vi "Cold_Flow_Test.vi"() -> ()   [LabVIEW 2024]
panel:
  in  "Stop":bool
  in  "Flow Time, ms":u32=1000
  out "Kerosene Valve":bool
  out "GOX Valve":bool
  in  "GOX Channel":tag="Dev1/port0/line1"
  in  "Kerosene Channel":tag="Dev1/port0/line3"
  # "Cold Flow Torch Igniter Test"
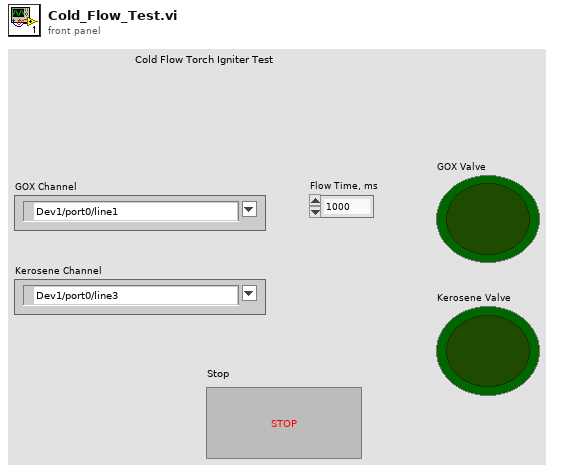
[diagram p1: front panel]
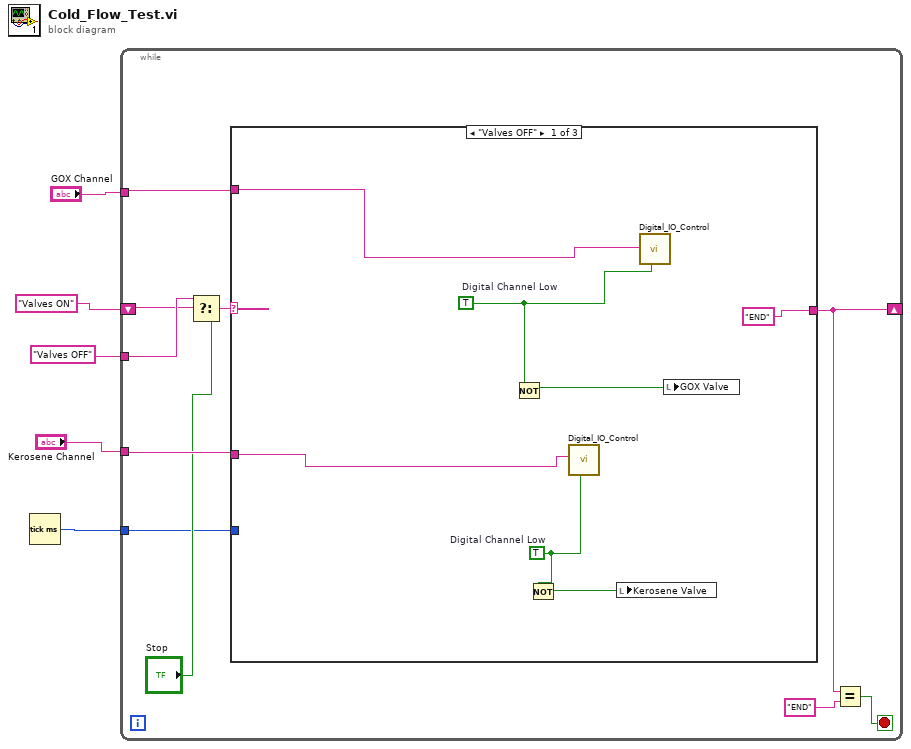
[diagram p0: block diagram]
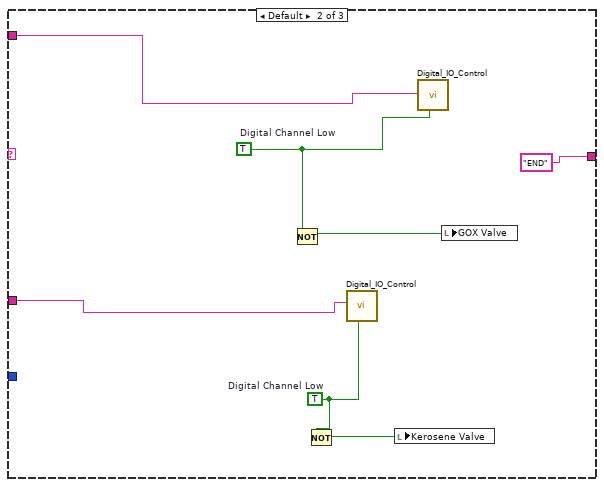
[diagram p2: hidden frame]
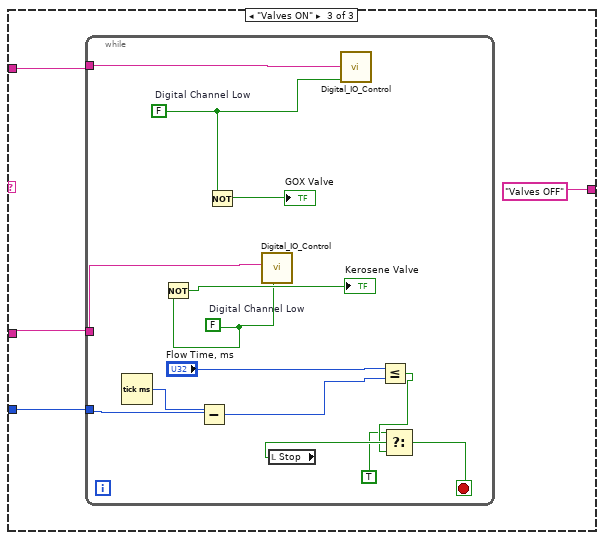
[diagram p3: hidden frame]
diagram:
  n1 = Tick Count (ms)() -> (millisecond timer value=w1:u32)
  n2 = while {
    tunnel: "Valves OFF" -> [w12]
    shift-right: [w8] -> _
    shift-left: "Valves ON" -> [w11]
    tunnel: "GOX Channel" -> [w15]
    tunnel: "Kerosene Channel" -> [w14]
    tunnel: w1 -> [w6]
    stop <- w9 stop-if-true
    n3 = Select(t=w12, s="Stop", f=w11) -> (s? t:f=w13:string)
    n4 = case shown="\"Valves OFF\"" w13 {
      tunnel: w15 -> [w20 w27 w33]
      tunnel: w14 -> [w19 w26 w32]
      tunnel: ["END" "END" "Valves OFF"] -> w8
      tunnel: w6 -> [_ _ w30]
      frame "Valves OFF" {
        w21 = TRUE  # Digital Channel Low
        w22 = TRUE  # Digital Channel Low
        n5 = Not(x=w22) -> (.not. x?=w18:bool)
        n6 = Not(x=w21) -> (.not. x?=w17:bool)
        n7 = call "Digital_IO_Control.vi"("Digital Channel High/Low (false : low)"=w21, "Digital Port Seclection"=w19) -> ()  [unwired: 6 in, 1 out]
        n8 = local write "Kerosene Valve"(w17) -> ()
        n9 = call "Digital_IO_Control.vi"("Digital Channel High/Low (false : low)"=w22, "Digital Port Seclection"=w20) -> ()  [unwired: 6 in, 1 out]
        n10 = local write "GOX Valve"(w18) -> ()
      }
      frame Default {
        w28 = TRUE  # Digital Channel Low
        w29 = TRUE  # Digital Channel Low
        n11 = Not(x=w29) -> (.not. x?=w25:bool)
        n12 = Not(x=w28) -> (.not. x?=w24:bool)
        n13 = call "Digital_IO_Control.vi"("Digital Channel High/Low (false : low)"=w28, "Digital Port Seclection"=w26) -> ()  [unwired: 6 in, 1 out]
        n14 = local write "Kerosene Valve"(w24) -> ()
        n15 = call "Digital_IO_Control.vi"("Digital Channel High/Low (false : low)"=w29, "Digital Port Seclection"=w27) -> ()  [unwired: 6 in, 1 out]
        n16 = local write "GOX Valve"(w25) -> ()
      }
      frame "Valves ON" {
        n17 = while {
          tunnel: w33 -> [w47]
          tunnel: w32 -> [w46]
          tunnel: w30 -> [w40]
          stop <- w34 stop-if-true
          w42 = FALSE  # Digital Channel Low
          w45 = FALSE  # Digital Channel Low
          n18 = Tick Count (ms)() -> (millisecond timer value=w39:u32)
          n19 = Not(x=w42) -> (.not. x?=→"Kerosene Valve":bool)
          n20 = Subtract(x=w39, y=w40) -> (x-y=w38:u32)
          n21 = Not(x=w45) -> (.not. x?=→"GOX Valve":bool)
          n22 = call "Digital_IO_Control.vi"("Digital Channel High/Low (false : low)"=w42, "Digital Port Seclection"=w46) -> ()  [unwired: 6 in, 1 out]
          n23 = local read "Stop"() -> (w41:bool)
          n24 = call "Digital_IO_Control.vi"("Digital Channel High/Low (false : low)"=w45, "Digital Port Seclection"=w47) -> ()  [unwired: 6 in, 1 out]
          n25 = Less Or Equal?(x="Flow Time, ms", y=w38) -> (x <= y?=w36:bool)
          n26 = Select(t=TRUE, s=w41, f=w36) -> (s? t:f=w34:bool)
        }
      }
    }
    n27 = Equal?(x=w8, y="END") -> (x = y?=w9:bool)
  }
